vi "Read Digital Input.vi"(8 "error in (no error)":errorcluster, 11 "VISA resource name":refnum<visa-resource-name>) -> (0 "error out":errorcluster, 2 "Digital Pins Input":bool[](array[boolean]), 3 "VISA resource name out":refnum<visa-resource-name>)   [LabVIEW 2021, in "Agilent N6900 N7900 Series.lvlib"]
doc: "Reads the digital values of the 7 digital pins (if they are configured to give digital input)"
uses:
  <instrlib>/Agilent N6900 N7900 Series/Agilent N6900 N7900 Series.lvlib
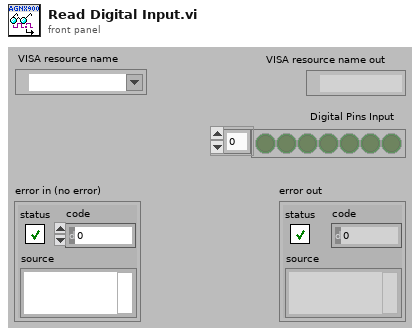
[diagram p1: front panel]
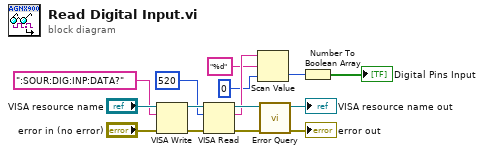
[diagram p0: block diagram]
diagram:
  n1 = VISA Write(VISA resource name="VISA resource name", write buffer=":SOUR:DIG:INP:DATA?", error in (no error)="error in (no error)") -> (VISA resource name out=w10:refnum<visa-resource-name>, error out=w11:errorcluster)  [unwired: 1 out]
  n2 = VISA Read(VISA resource name=w10, byte count=u32 520, error in (no error)=w11) -> (VISA resource name out=w12:refnum<visa-resource-name>, read buffer=w6:string, error out=w13:errorcluster)  [unwired: 1 out]
  n3 = Scan Value(string=w6, format string="%d", default (0 dbl)=0) -> (value=w4:i32)  [unwired: 1 out]
  n4 = call <instrlib>:"Error Query.vi"("error in (no error)"=w13, "VISA resource name"=w12) -> ("error out"=→"error out":errorcluster, "VISA resource name out"=→"VISA resource name out":refnum<visa-resource-name>)  [unwired: 6 in, 2 out]
  n5 = Number To Boolean Array(number=w4) -> (Boolean array=→"Digital Pins Input":bool[])
